vi "Configure Date And Time.vi"(7 "Unit Address (1)":i16=1, 8 "error in (no error)":errorcluster {"code" format="%.0x"}, 10 "Input Array (0; 0; 0; 1; 1; 2004)":i16[](array[numeric])=[0, 0, 0, 1, 1, 2004], 11 "VISA resource name":refnum<visa-resource-name>) -> (0 "error out":errorcluster {"code" format="%.0x"}, 3 "VISA resource name out":refnum<visa-resource-name>)   [LabVIEW 2010]
doc: "This VI gets or sets date and time."
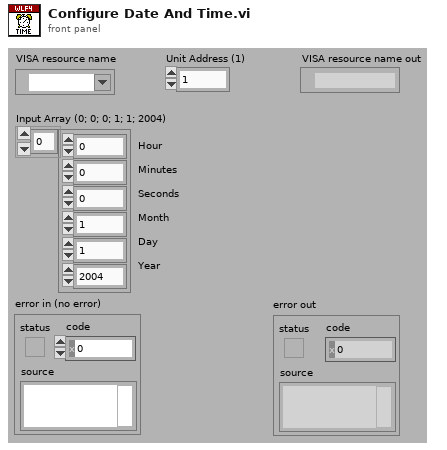
[diagram p1: front panel]
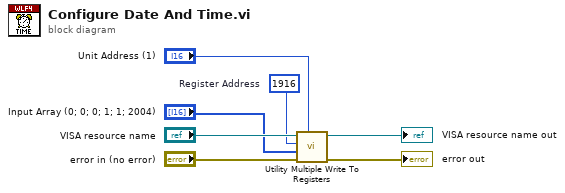
[diagram p0: block diagram]
diagram:
  w1 = u16 1916  # Register Address
  n1 = call "Utility Multiple Write To Registers.vi"("Unit Address (1)"="Unit Address (1)", "error in (no error)"="error in (no error)", "Array Of Data"="Input Array (0; 0; 0; 1; 1; 2004)", "Register Address (0)"=w1, "VISA resource name"="VISA resource name") -> ("error out"=→"error out":errorcluster, "VISA resource name out"=→"VISA resource name out":refnum<visa-resource-name>)  [unwired: 5 in]
